vi "Test ModuleInterface API.vi"() -> ()   [LabVIEW 2018]
doc: "ModuleInterface API Tester."
uses:
  <vilib>/Utility/error.llb/DialogType.ctl
  ModuleInterface.lvlib
  MainInterface/MainInterface.lvlib
panel:
  in  "Enable Item":bool
  in  "Item Name":string
  in  "Disable Item":bool
  in  "Get Module ID List":bool
  in  "Get Module Name":bool
  in  "模块名称":string="测试工作站"
  in  "枚举":enum16{"Station", "Function Block"}(ring)
  out "last error":errorcluster
  in  "Show Diagram on Init":bool
  in  "Run as Singleton?":bool
  in  "Show Block Diagram":bool
  in  "Refresh Modules":bool
  out "Active Modules":string[](array[string])
  in  "Stop Module":bool
  in  "Select Module":i32(ring)=-1 caption="Select Module\nTo send Request to" items=["All"=-1]
  in  "Run New Module":bool
  in  "Hide Module Panel":bool
  in  "Show Module Panel":bool
  out "Status":string
  # "This VI tests the API for the Module."
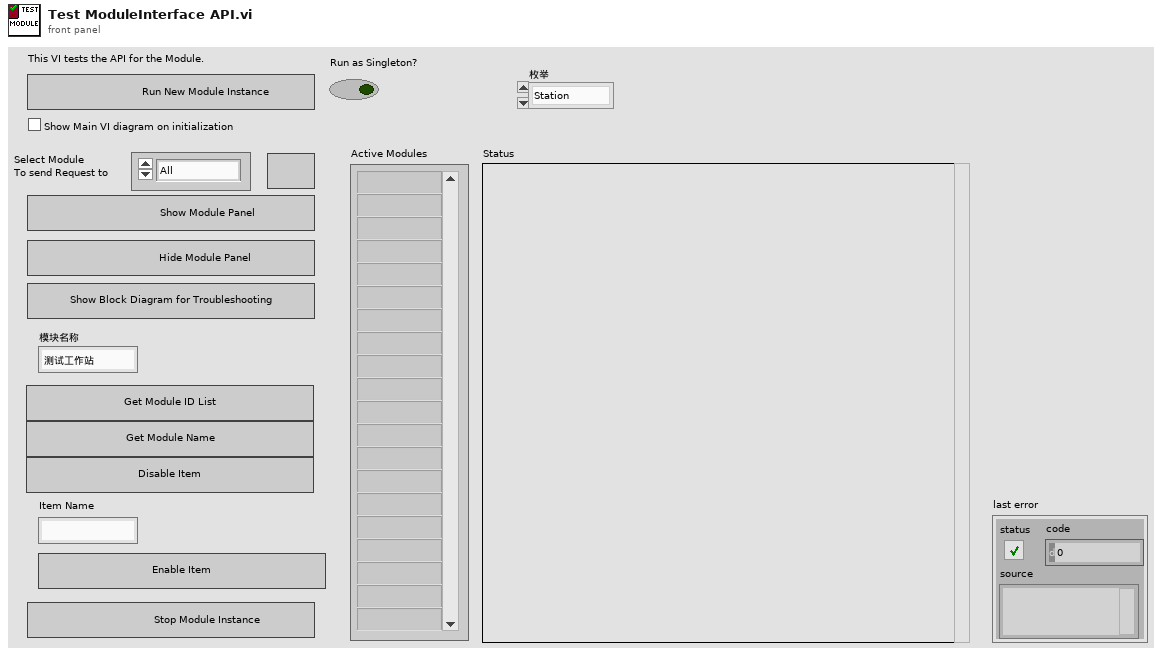
[diagram p1: front panel]
types:
  T1 = typedef "ModuleInterface.lvlib/Broadcast Events--cluster.ctl" = cluster{"Module Did Init":refnum<user-event>, "Status Updated":refnum<user-event>, "Error Reported":refnum<user-event>, "Module Did Stop":refnum<user-event>, "Update Module Execution Status":refnum<user-event>, "Function Selected":refnum<user-event>, "Window Size Changed":refnum<user-event>}
  T2 = typedef "DialogType.ctl" = u16
  T3 = typedef "ModuleInterface.lvlib/ModuleDefinition.ctl" = cluster{"模块名称":string, "项定义":T4[]}
  T4 = typedef "ModuleInterface.lvlib/FunctionItem.ctl" = cluster{"项名":string, "符号图形路径":path}
  T5 = typedef "LVRectTypeDef.ctl" = cluster{"Left":i16, "Top":i16, "Right":i16, "Bottom":i16}
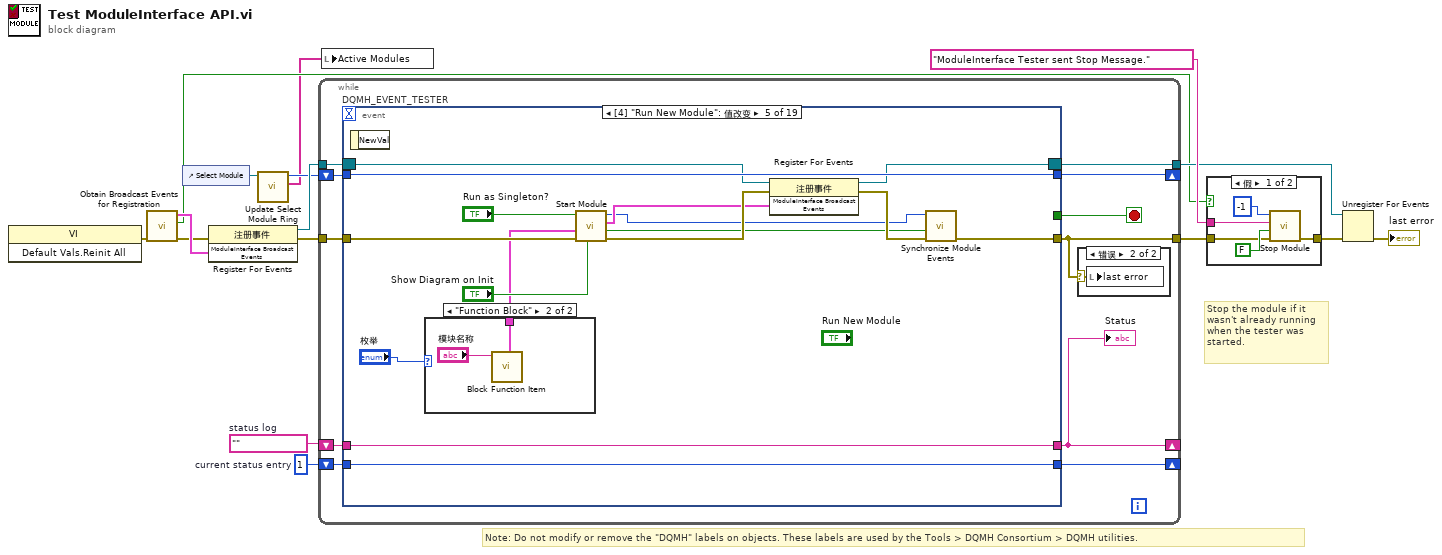
[diagram p0: block diagram]
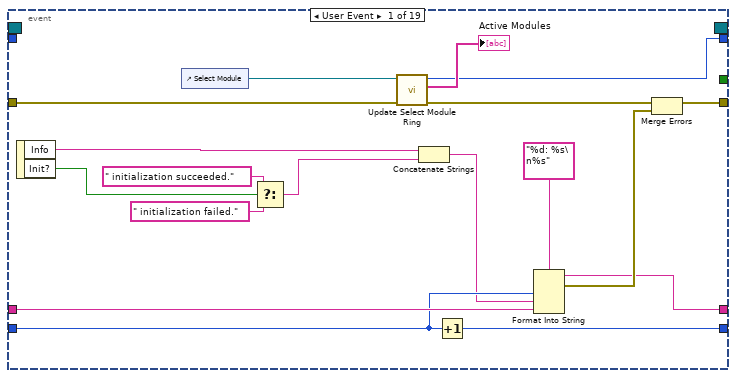
[diagram p4: hidden frame]
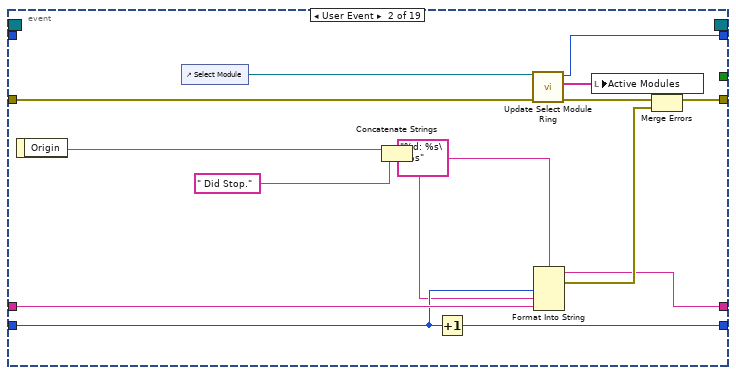
[diagram p5: hidden frame]
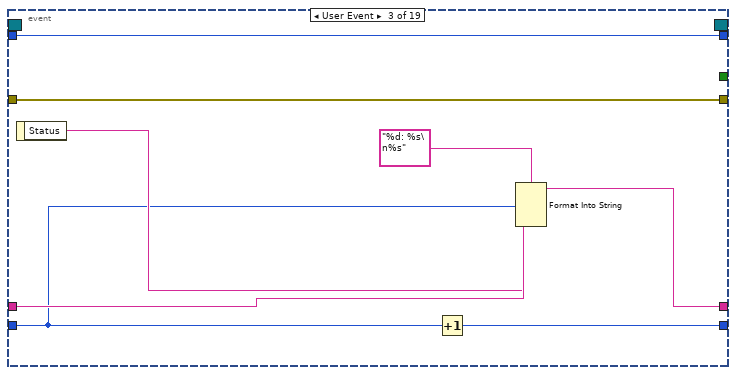
[diagram p6: hidden frame]
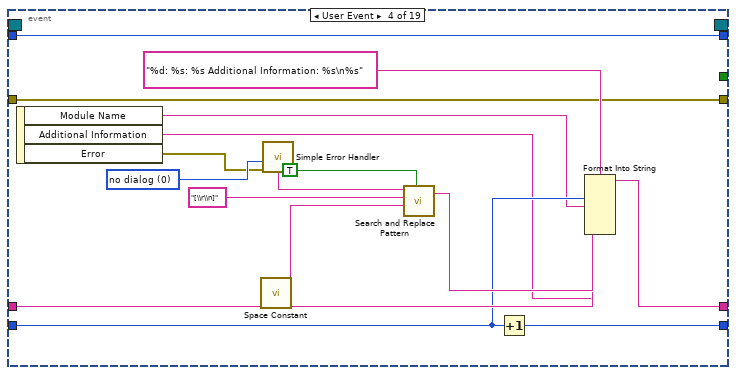
[diagram p7: hidden frame]
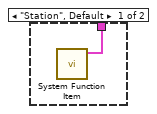
[diagram p8: hidden frame]
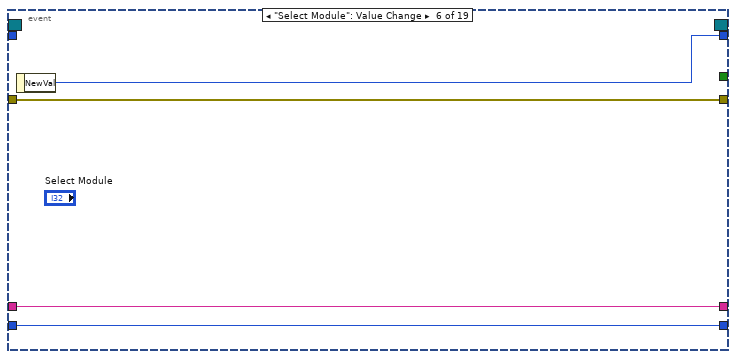
[diagram p9: hidden frame]
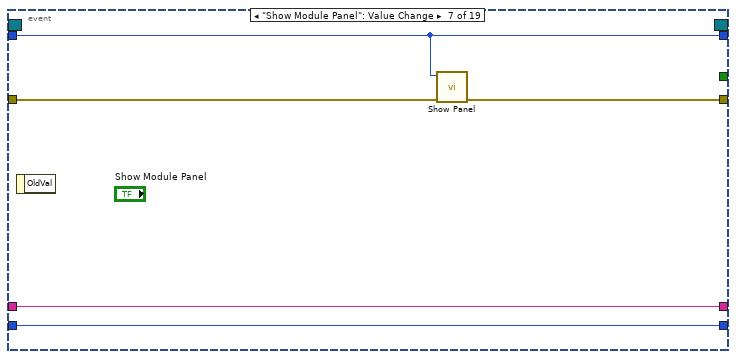
[diagram p10: hidden frame]
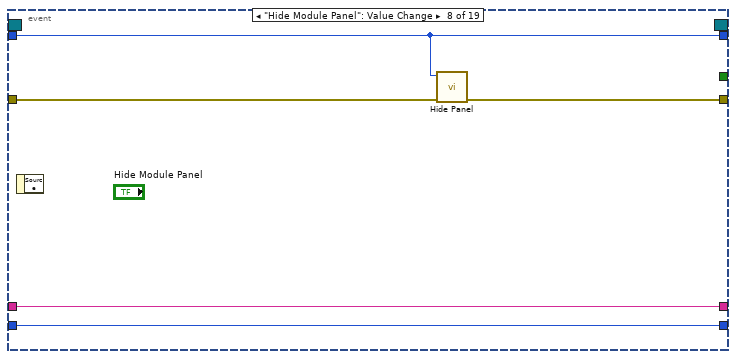
[diagram p11: hidden frame]
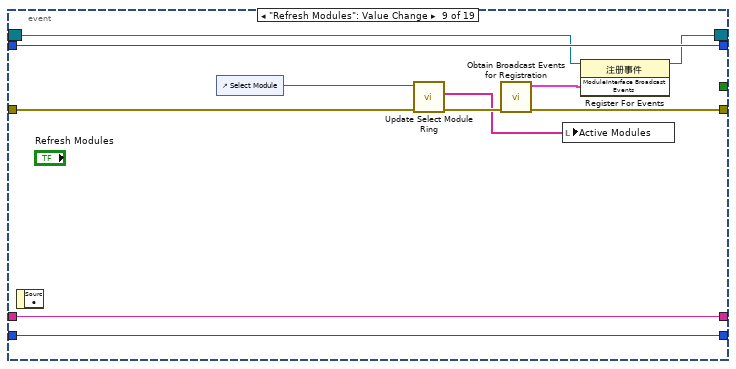
[diagram p12: hidden frame]
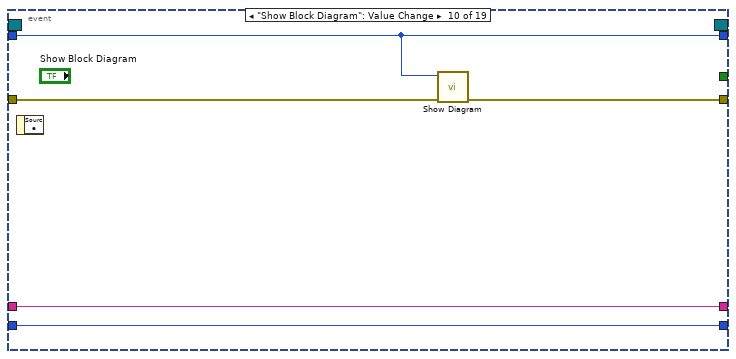
[diagram p13: hidden frame]
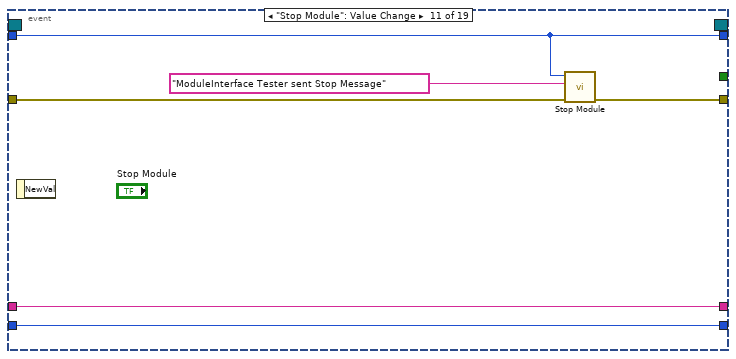
[diagram p14: hidden frame]
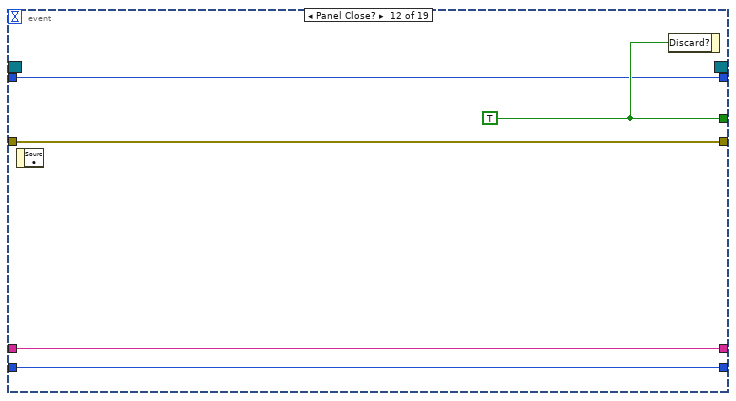
[diagram p15: hidden frame]
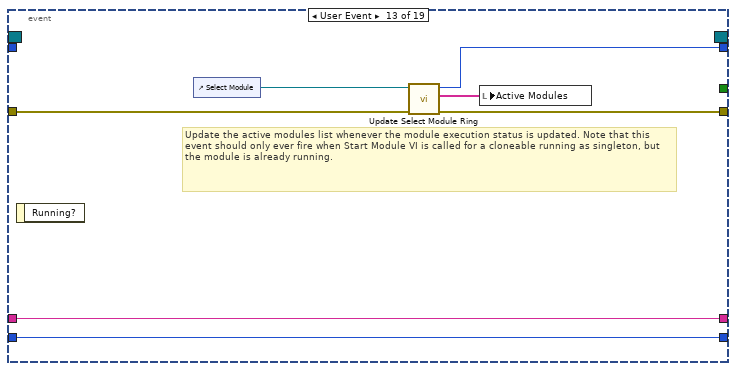
[diagram p16: hidden frame]
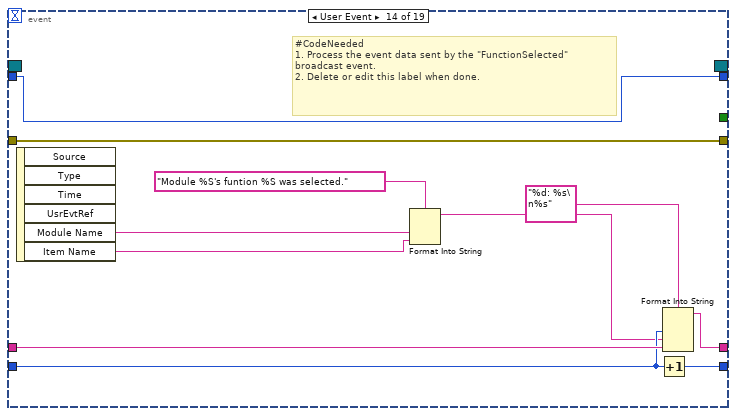
[diagram p17: hidden frame]
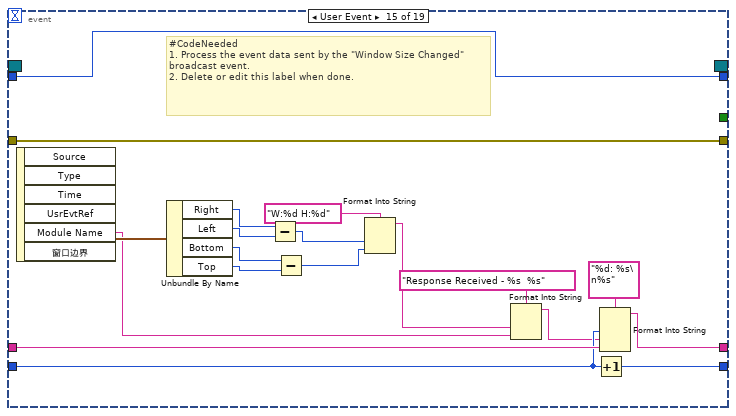
[diagram p18: hidden frame]
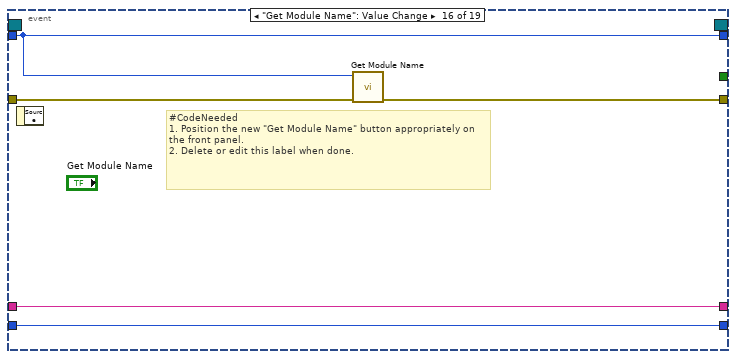
[diagram p19: hidden frame]
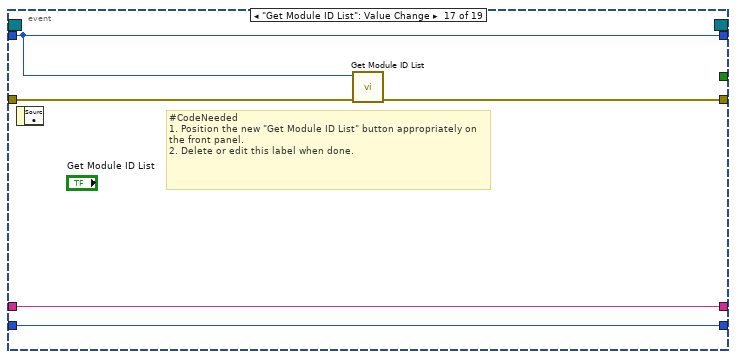
[diagram p20: hidden frame]
diagram:
  w13 = 1  # current status entry
  w14 = ""  # status log
  # "Stop the module if it wasn't already running when the tester was started."
  # "Note: Do not modify or remove the \"DQMH\" labels on objects. These labels are used by the Tools > DQMH Consortium > DQMH utilities."
  n1 = invoke class="VI" method="Default Vals.Reinit All"() -> (error out=w8:errorcluster)  [unwired: 3 in, 2 out]
  n2 = call "Obtain Broadcast Events for Registration.vi"("error in"=w8) -> ("error out"=w7:errorcluster, "Already running?"=w6:bool, "ModuleInterface Broadcast Events"=w12:T1)  [unwired: 8 in]
  n3 = control-ref of="Select Module"() -> (w3:refnum<vi>)
  n4 = register-events(error in=w7, w12) -> (reference out=w16:refnum<event-registration>, error out=w11:errorcluster)  [unwired: 1 in]
  n5 = call "Update Select Module Ring.vi"("Select Module Ring Ref"=w3) -> ("Active Modules (Array)"=w1:string[], "New Module Ring Value"=w2:i32)  [unwired: 8 in, 1 out]
  n6 = while {
    tunnel: w16 -> [w27]
    tunnel: [w18] -> w5
    tunnel: w11 -> [w26]
    shift-right: [w22] -> _
    shift-left: w14 -> [w24]
    shift-right: [w23] -> _
    shift-left: w13 -> [w25]
    shift-right: [w20] -> _
    shift-left: w2 -> [w21]
    tunnel: [w19] -> w9
    stop <- w17 stop-if-true
    n7 = event "DQMH_EVENT_TESTER" shown="[4] \"Run New Module\": 值改变" {
      selector: w27 -> [_ _ _ _ w95 _ _ _ w124 _ _ _ _ _ _ _ _ _ _]
      dyn-events: [_ _ _ _ w94 _ _ _ w123 _ _ _ _ _ _ _ _ _ _] -> w19
      timeout: _ -> [_ _ _ _ _ _ _ _ _ _ _ _ _ _ _ _ _ _ _]
      tunnel: [_ _ _ _ _ _ _ _ _ _ _ w145 _ _ _ _ _ _ _] -> w17
      tunnel: [w36 w53 w69 w73 w93 w108 w112 w117 w120 w131 w136 w144 w148 w163 w182 w183 w188 w194 w200] -> w18
      tunnel: w26 -> [w38 w55 w69 w73 w96 w108 w113 w118 w125 w134 w137 w144 w149 w163 w182 w187 w192 w198 w204]
      tunnel: w25 -> [w43 w58 w62 w76 w98 w106 w110 w115 w128 w132 w139 w142 w151 w159 w178 w185 w190 w196 w202]
      tunnel: w24 -> [w44 w59 w65 w77 w99 w107 w111 w116 w129 w133 w140 w143 w152 w161 w180 w186 w191 w197 w203]
      tunnel: [w41 w56 w66 w75 w99 w107 w111 w116 w129 w133 w140 w143 w152 w160 w179 w186 w191 w197 w203] -> w22
      tunnel: [w42 w57 w68 w74 w98 w106 w110 w115 w128 w132 w139 w142 w151 w158 w177 w185 w190 w196 w202] -> w23
      tunnel: w21 -> [_ _ w63 w85 w97 _ w109 w114 w127 w130 w138 w141 _ w162 w181 w184 w189 w195 w201]
      tunnel: [w33 w50 w63 w85 w97 w105 w109 w114 w127 w130 w138 w141 w147 w162 w181 w184 w189 w195 w201] -> w20
      event User Event {
        n8 = event-data() -> ("Info"=w40:string, "Init?"=w30:bool)  [unwired: 1 in]
        n9 = control-ref of="Select Module"() -> (w35:refnum<vi>)
        n10 = Select(t=" initialization succeeded.", s=w30, f=" initialization failed.") -> (s? t:f=w29:string)
        n11 = call "Update Select Module Ring.vi"("error in"=w38, "Select Module Ring Ref"=w35) -> ("error out"=w37:errorcluster, "Active Modules (Array)"=→"Active Modules":string[], "New Module Ring Value"=w33:i32)  [unwired: 7 in]
        n12 = Concatenate Strings(w40, w29) -> (w39:string)
        n13 = Increment(x=w43) -> (x+1=w42:i32)
        n14 = Format Into String(format string="%d: %s\n%s", w43, w39, w44) -> (resulting string=w41:string, error out=w46:errorcluster)  [unwired: 2 in]
        n15 = Merge Errors(w37, w46) -> (w36:errorcluster)
      }
      event User Event {
        n16 = event-data() -> ("Origin"=w48:string)  [unwired: 1 in]
        n17 = control-ref of="Select Module"() -> (w52:refnum<vi>)
        n18 = Concatenate Strings(w48, " Did Stop.") -> (w47:string)
        n19 = Increment(x=w58) -> (x+1=w57:i32)
        n20 = call "Update Select Module Ring.vi"("error in"=w55, "Select Module Ring Ref"=w52) -> ("error out"=w54:errorcluster, "Active Modules (Array)"=w51:string[], "New Module Ring Value"=w50:i32)  [unwired: 7 in]
        n21 = Format Into String(format string="%d: %s\n%s", w58, w47, w59) -> (resulting string=w56:string, error out=w61:errorcluster)  [unwired: 2 in]
        n22 = local write "Active Modules"(w51) -> ()
        n23 = Merge Errors(w54, w61) -> (w53:errorcluster)
      }
      event User Event {
        n24 = event-data() -> ("Status"=w64:string)  [unwired: 1 in]
        n25 = Increment(x=w62) -> (x+1=w68:i32)
        n26 = Format Into String(format string="%d: %s\n%s", w62, w64, w65) -> (resulting string=w66:string)  [unwired: 2 in, 1 out]
      }
      event User Event {
        w78 = T2 0 items=["no dialog", "OK message", "continue or stop message", "OK message + warnings", "continue/stop + warnings"] ("type of dialog (OK msg:1)")
        n27 = event-data() -> ("Module Name"=w72:string, "Additional Information"=w71:string, "Error"=w70:errorcluster)  [unwired: 1 in]
        n28 = call <vilib>:"Space Constant.vi"() -> ("String"=w82:string)
        n29 = call <vilib>:"Simple Error Handler.vi"("type of dialog (OK msg:1)"=w78, "error in (no error)"=w70) -> ("message"=w79:string)  [unwired: 3 in, 4 out]
        n30 = call <vilib>:"Search and Replace Pattern.vi"("string"=w79, "regular expression (\"\")"="[\\r\\n]" ("regular expression (\"\")"), "replace string (\"\")"=w82, "replace all? (F)"=TRUE ("replace all CR/LF with spaces")) -> ("result string"=w80:string)  [unwired: 1 in, 1 out]
        n31 = Increment(x=w76) -> (x+1=w74:i32)
        n32 = Format Into String(format string="%d: %s: %s Additional Information: %s\n%s", w76, w72, w80, w71, w77) -> (resulting string=w75:string)  [unwired: 2 in, 1 out]
      }
      event "Run New Module": Value Change {
        n33 = event-data() -> ()  [unwired: 1 in, 1 out]
        n34 = case shown="\"Function Block\"" "枚举" {
          tunnel: [w102 w104] -> w87
          frame "Station", Default {
            n35 = call "System Function Item.vi"() -> ("模块定义"=w102:T3)  [unwired: 11 in]
          }
          frame "Function Block" {
            n36 = call "Block Function Item.vi"("模块名称"="模块名称") -> ("模块定义"=w104:T3)  [unwired: 10 in]
          }
        }
        n37 = call "Start Module.vi"("Show Main VI Diagram on Init (F)"="Show Diagram on Init", "error in"=w96, "模块定义"=w87, "Run as Singleton? (F)"="Run as Singleton?") -> ("error out"=w100:errorcluster, "Wait for Event Sync?"=w92:bool, "ModuleInterface Broadcast Events"=w91:T1, "Module ID"=w88:i32)  [unwired: 4 in]
        n38 = register-events(reference=w95, error in=w100, w91) -> (reference out=w94:refnum<event-registration>, error out=w101:errorcluster)
        n39 = call "Synchronize Module Events.vi"("error in"=w101, "Wait for Event Sync?"=w92, "Module ID in"=w88) -> ("error out"=w93:errorcluster)  [unwired: 7 in, 1 out]
      }
      event "Select Module": Value Change {
        n40 = event-data() -> ("NewVal"=w105:i32)  [unwired: 1 in]
      }
      event "Show Module Panel": Value Change {
        n41 = event-data() -> ()  [unwired: 1 in, 1 out]
        n42 = call "Show Panel.vi"("error in"=w113, "Module ID"=w109) -> ("error out"=w112:errorcluster)  [unwired: 9 in]
      }
      event "Hide Module Panel": Value Change {
        n43 = event-data() -> ()  [unwired: 1 in, 1 out]
        n44 = call "Hide Panel.vi"("error in"=w118, "Module ID"=w114) -> ("error out"=w117:errorcluster)  [unwired: 9 in]
      }
      event "Refresh Modules": Value Change {
        n45 = event-data() -> ()  [unwired: 1 in, 1 out]
        n46 = control-ref of="Select Module"() -> (w126:refnum<vi>)
        n47 = call "Update Select Module Ring.vi"("error in"=w125, "Select Module Ring Ref"=w126) -> ("error out"=w121:errorcluster, "Active Modules (Array)"=w119:string[])  [unwired: 7 in, 1 out]
        n48 = call "Obtain Broadcast Events for Registration.vi"("error in"=w121) -> ("error out"=w120:errorcluster, "ModuleInterface Broadcast Events"=w122:T1)  [unwired: 8 in, 1 out]
        n49 = local write "Active Modules"(w119) -> ()
        n50 = register-events(reference=w124, w122) -> (reference out=w123:refnum<event-registration>)  [unwired: 1 in, 1 out]
      }
      event "Show Block Diagram": Value Change {
        n51 = event-data() -> ()  [unwired: 1 in, 1 out]
        n52 = call "Show Diagram.vi"("error in"=w134, "Module ID"=w130) -> ("error out"=w131:errorcluster)  [unwired: 9 in]
      }
      event "Stop Module": Value Change {
        n53 = event-data() -> ()  [unwired: 1 in, 1 out]
        n54 = call "Stop Module.vi"("error in"=w137, "Origin"="ModuleInterface Tester sent Stop Message", "Module ID"=w138) -> ("error out"=w136:errorcluster)  [unwired: 8 in]
      }
      event Panel Close? {
        w145 = TRUE ("Discard?")
        n55 = event-data() -> ()  [unwired: 1 in, 1 out]
        n56 = event-data("Discard?"=w145) -> ()  [unwired: 1 in, 1 out]
      }
      event User Event {
        # "Update the active modules list whenever the module execution status is updated. Note that this event should only ever fire when Start Module VI is called for a cloneable running as singleton, but the module is already running."
        n57 = event-data() -> ()  [unwired: 1 in, 1 out]
        n58 = control-ref of="Select Module"() -> (w150:refnum<vi>)
        n59 = call "Update Select Module Ring.vi"("error in"=w149, "Select Module Ring Ref"=w150) -> ("error out"=w148:errorcluster, "Active Modules (Array)"=w146:string[], "New Module Ring Value"=w147:i32)  [unwired: 7 in]
        n60 = local write "Active Modules"(w146) -> ()
      }
      event User Event {
        # "#CodeNeeded\n1. Process the event data sent by the \"FunctionSelected\" broadcast event.\n2. Delete or edit this label when done."
        n61 = event-data() -> ("Module Name"=w154:string, "Item Name"=w153:string)  [unwired: 1 in, 4 out]
        n62 = Format Into String(format string="Module %S's funtion %S was selected." ("格式字符串"), w154, w153) -> (resulting string=w156:string)  [unwired: 2 in, 1 out]
        n63 = Increment(x=w159) -> (x+1=w158:i32)
        n64 = Format Into String(format string="%d: %s\n%s", w159, w156, w161) -> (resulting string=w160:string)  [unwired: 2 in, 1 out]
      }
      event User Event {
        # "#CodeNeeded\n1. Process the event data sent by the \"Window Size Changed\" broadcast event.\n2. Delete or edit this label when done."
        n65 = event-data() -> ("Module Name"=w164:string, "窗口边界"=w166:T5)  [unwired: 1 in, 4 out]
        n66 = Unbundle By Name(w166) -> ("Right"=w169:i16, "Left"=w170:i16, "Bottom"=w171:i16, "Top"=w172:i16)
        n67 = Subtract(x=w169, y=w170) -> (x-y=w168:i16)
        n68 = Subtract(x=w171, y=w172) -> (x-y=w173:i16)
        n69 = Format Into String(format string="W:%d H:%d" ("格式字符串"), w168, w173) -> (resulting string=w165:string)  [unwired: 2 in, 1 out]
        n70 = Format Into String(format string="Response Received - %s  %s", w165, w164) -> (resulting string=w174:string)  [unwired: 2 in, 1 out]
        n71 = Increment(x=w178) -> (x+1=w177:i32)
        n72 = Format Into String(format string="%d: %s\n%s", w178, w174, w180) -> (resulting string=w179:string)  [unwired: 2 in, 1 out]
      }
      event "Get Module Name": Value Change {
        # "#CodeNeeded\n1. Position the new \"Get Module Name\" button appropriately on the front panel.\n2. Delete or edit this label when done."
        n73 = event-data() -> ()  [unwired: 1 in, 1 out]
        n74 = call "Get Module Name.vi"("error in"=w187, "Module ID"=w184) -> ("error out"=w183:errorcluster)  [unwired: 6 in, 3 out]
      }
      event "Get Module ID List": Value Change {
        # "#CodeNeeded\n1. Position the new \"Get Module ID List\" button appropriately on the front panel.\n2. Delete or edit this label when done."
        n75 = event-data() -> ()  [unwired: 1 in, 1 out]
        n76 = call "Get Module ID List.vi"("error in"=w192, "Module ID"=w189) -> ("error out"=w188:errorcluster)  [unwired: 7 in, 2 out]
      }
      event "Disable Item": Value Change {
        # "#CodeNeeded\n1. Position the new \"Disable Item\" button appropriately on the front panel.\n2. Delete or edit this label when done."
        n77 = event-data() -> ()  [unwired: 1 in, 1 out]
        n78 = call "Disable Item.vi"("error in"=w198, "Item Name"="Item Name", "Module ID"=w195) -> ("error out"=w194:errorcluster)  [unwired: 8 in]
      }
      event "Enable Item": Value Change {
        n79 = event-data() -> ()  [unwired: 1 in, 1 out]
        n80 = local read "Item Name"() -> (w199:string)
        n81 = call "Enable Item.vi"("error in"=w204, "Item Name"=w199, "Module ID"=w201) -> ("error out"=w200:errorcluster)  [unwired: 8 in]
      }
    }
    "Status" <- w22
    n82 = case shown="错误" w18 {
      selector: w18 -> [_ w28]
      frame No Error {
      }
      frame Error {
        n83 = local write "last error"(w28) -> ()
      }
    }
  }
  n84 = local write "Active Modules"(w1) -> ()
  n85 = case shown="假" w6 {
    tunnel: [w209 w210] -> w15
    tunnel: "ModuleInterface Tester sent Stop Message." ("Origin") -> [w208 _]
    tunnel: w5 -> [w205 w210]
    frame False {
      n86 = call "Stop Module.vi"("error in"=w205, "Wait for Module to stop? (F)"=FALSE ("Wait for Module to stop?"), "Origin"=w208, "Module ID"=-1 ("Stop all")) -> ("error out"=w209:errorcluster)  [unwired: 7 in]
    }
    frame True {
    }
  }
  n87 = Unregister For Events(event registration refnum=w9, error in=w15) -> (error out=→"last error":errorcluster)
